vi "create buffer queue.vi"(8 "error in (no error)":errorcluster, 11 "Sink-Console in":refnum<class "Sink-Console.lvclass">) -> (0 "error out":errorcluster, 3 "Sink-Console out":refnum<class "Sink-Console.lvclass">)   [LabVIEW 2019, in "TSC Event Logger.lvlib" / "Sink-Console.lvclass"]
doc: "create a buffer queue for the console sink.\n\n<b>Code Developed By:</b>\nTechnology Service Corporation\nBloomington, IN 47403\nwww.tsc.com/atcs\n\nDeveloper:\nDaniel Coons"
uses:
  Sink-Console.lvclass
  Sink-Console.lvclass/Sink-Console.ctl
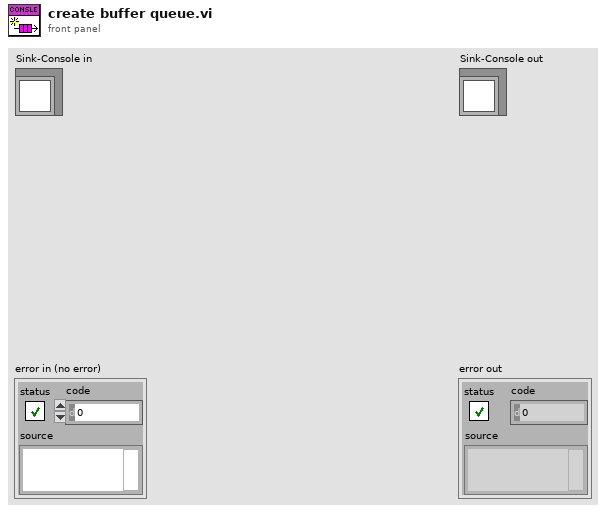
[diagram p1: front panel]
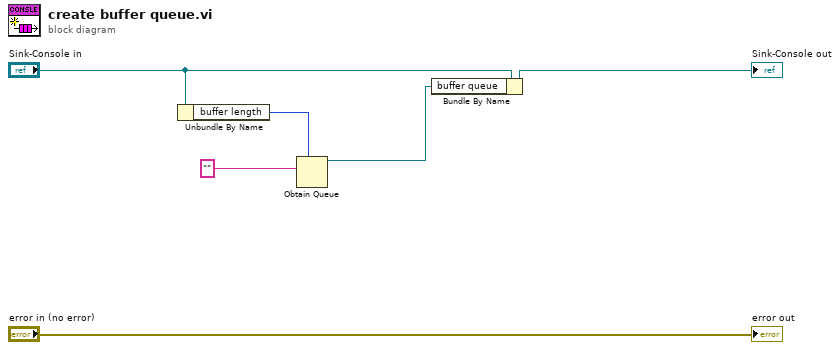
[diagram p0: block diagram]
diagram:
  n1 = Unbundle By Name("Sink-Console in") -> ("buffer length"=w3:i32)
  n2 = Obtain Queue(max queue size (-1, unlimited)=w3, element data type="") -> (queue out=w1:refnum<queue>)  [unwired: 3 in, 2 out]
  n3 = Bundle By Name(cluster="Sink-Console in", "buffer queue"=w1) -> (→"Sink-Console out":refnum<class "Sink-Console.lvclass">)
  "error out" <- "error in (no error)"
